vi "Next Pose.vi"(7 "Step":dbl=25.0, 8 "Start":T1 format="%.3f", 11 "Goal":T1 format="%.3f") -> (0 "Pose":T1 format="%.3f", 3 "At Goal":bool)   [LabVIEW 2013]
uses:
  <vilib>/Analysis/Matrix/Datatypes/RealMatrix.ctl
  <vilib>/Analysis/baseanly.llb/Real Dot Product.vi
  <vilib>/Analysis/Matrix/Numeric/Conversions/Array To Matrix - RA2.vi
  <vilib>/Analysis/NI_AALBase.lvlib
  <vilib>/Analysis/Matrix/NI_Matrix.lvlib
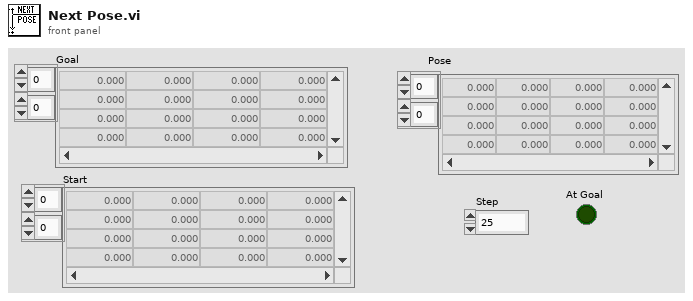
[diagram p1: front panel]
types:
  T1 = typedef "NI_Matrix.lvlib/RealMatrix.ctl" = dbl[][]
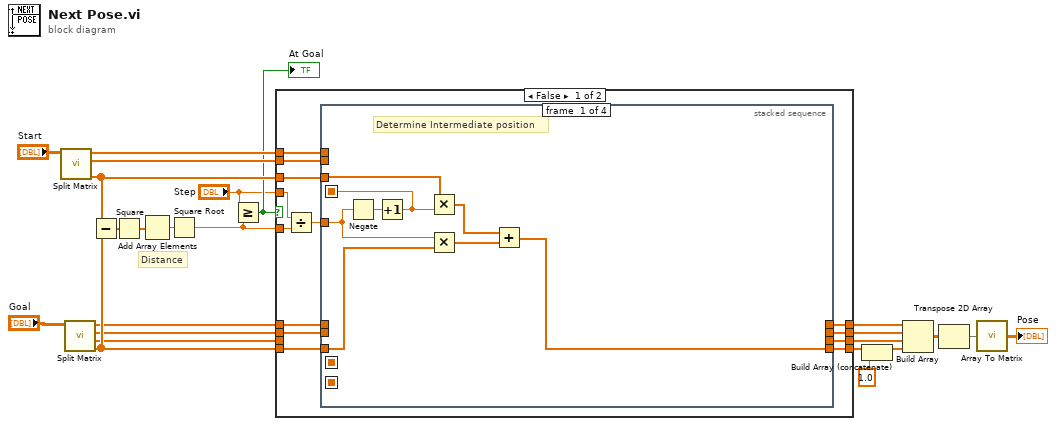
[diagram p0: block diagram]
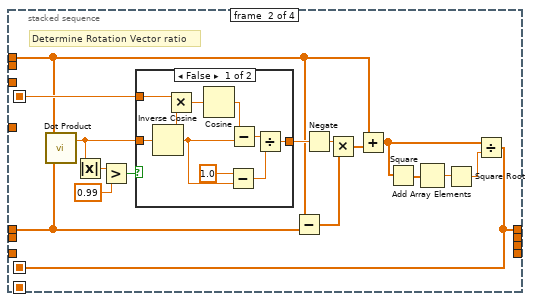
[diagram p2: hidden frame]
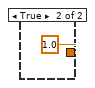
[diagram p3: hidden frame]
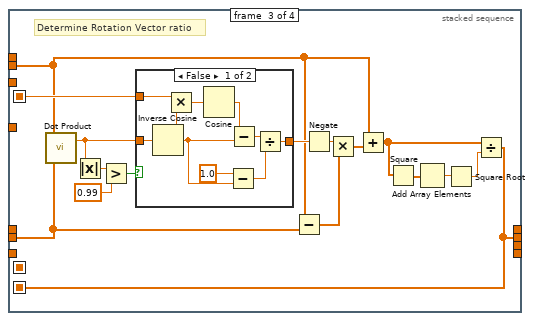
[diagram p4: hidden frame]
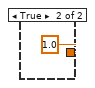
[diagram p5: hidden frame]
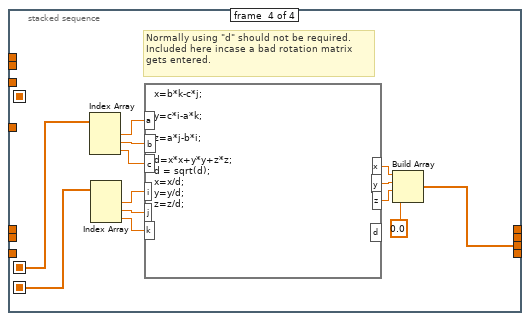
[diagram p6: hidden frame]
diagram:
  # "Distance"
  n1 = call "Split Matrix.vi"("Current"="Start") -> ("Position"=w21:dbl[], "Approach"=w17:dbl[], "Normal"=w18:dbl[])  [unwired: 7 in, 1 out]
  n2 = call "Split Matrix.vi"("Current"="Goal") -> ("Position"=w20:dbl[], "Tangent"=w14:dbl[], "Approach"=w15:dbl[], "Normal"=w16:dbl[])  [unwired: 7 in]
  n3 = Subtract ("Subtract.vi")(x=w21, y=w20) -> (x-y=w22:dbl[])
  n4 = Square(x=w22) -> (x^2=w23:dbl[])
  n5 = Add Array Elements(numeric array=w23) -> (sum=w24:dbl)
  n6 = Square Root(x=w24) -> (sqrt(x)=w4:dbl)
  n7 = Greater Or Equal?(x="Step", y=w4) -> (x >= y?=w6:bool)
  "At Goal" <- w6
  n8 = case shown="False" w6 {
    tunnel: w4 -> [w37 _]
    tunnel: "Step" -> [w35 _]
    tunnel: w20 -> [w34 w114]
    tunnel: w21 -> [w33 _]
    tunnel: [w32 w114] -> w2
    tunnel: w18 -> [w31 _]
    tunnel: w17 -> [w30 _]
    tunnel: w16 -> [w29 w113]
    tunnel: w15 -> [w28 w112]
    tunnel: [w27 w113] -> w11
    tunnel: [w26 w112] -> w12
    tunnel: w14 -> [_ w111]
    tunnel: [w25 w111] -> w13
    frame False {
      n9 = Divide(x=w35, y=w37) -> (x/y=w36:dbl)
      n10 = stacked-sequence {
        seq-local: [w39 _ _ _] -> [_ w61 w87 _]
        seq-local: [_ w46 _ _] -> [_ _ _ w98]
        seq-local: [_ _ w72 _] -> [_ _ _ w99]
        tunnel: w36 -> [w43 _ _ _]
        tunnel: w34 -> [w45 _ _ _]
        tunnel: w33 -> [w44 _ _ _]
        tunnel: [w38 _ _ _] -> w32
        tunnel: w31 -> [_ w51 _ _]
        tunnel: w30 -> [_ _ w73 _]
        tunnel: w29 -> [_ w56 _ _]
        tunnel: w28 -> [_ _ w74 _]
        tunnel: [_ w46 _ _] -> w27
        tunnel: [_ _ w72 _] -> w26
        tunnel: [_ _ _ w107] -> w25
        frame #0 {
          # "Determine Intermediate position"
          n11 = Negate(x=w43) -> (-x=w40:dbl)
          n12 = Increment(x=w40) -> (x+1=w39:dbl)
          n13 = Multiply ("Multiply.vi")(x=w44, y=w39) -> (x*y=w42:dbl[])
          n14 = Multiply ("Multiply.vi")(x=w43, y=w45) -> (x*y=w41:dbl[])
          n15 = Add ("Add.vi")(x=w42, y=w41) -> (x+y=w38:dbl[])
        }
        frame #1 {
          # "Determine Rotation Vector ratio"
          n16 = call-poly <vilib>:"Dot Product.vi"("Y Vector"=w56, "X Vector"=w51) -> ("X * Y"=w60:dbl)  [unwired: 1 out]
          n17 = Absolute Value(x=w60) -> (abs(x)=w59:dbl)
          n18 = Greater?(x=w59, y=0.99) -> (0:w57:bool)
          n19 = case shown="False" w57 {
            tunnel: w61 -> [w70 _]
            tunnel: w60 -> [w69 _]
            tunnel: [w62 1.0] -> w55
            frame False {
              n20 = Inverse Cosine(1:w69) -> (0:w66:dbl)
              n21 = Multiply(x=w70, y=w66) -> (x*y=w68:dbl)
              n22 = Cosine(x=w68) -> (cos(x)=w67:dbl)
              n23 = Subtract(x=1.0, y=w66) -> (x-y=w63:dbl)
              n24 = Subtract(x=w67, y=w66) -> (x-y=w64:dbl)
              n25 = Divide(x=w64, y=w63) -> (x/y=w62:dbl)
            }
            frame True {
            }
          }
          n26 = Subtract(x=w51, y=w56) -> (x-y=w54:dbl[])
          n27 = Negate(x=w55) -> (-x=w53:dbl)
          n28 = Multiply(x=w53, y=w54) -> (x*y=w52:dbl[])
          n29 = Add(x=w51, y=w52) -> (x+y=w47:dbl[])
          n30 = Square(x=w47) -> (x^2=w50:dbl[])
          n31 = Add Array Elements(numeric array=w50) -> (sum=w49:dbl)
          n32 = Square Root(x=w49) -> (sqrt(x)=w48:dbl)
          n33 = Divide(x=w47, y=w48) -> (x/y=w46:dbl[])
        }
        frame #2 {
          # "Determine Rotation Vector ratio"
          n34 = call-poly <vilib>:"Dot Product.vi"("Y Vector"=w74, "X Vector"=w73) -> ("X * Y"=w86:dbl)  [unwired: 1 out]
          n35 = Absolute Value(x=w86) -> (abs(x)=w85:dbl)
          n36 = Greater?(x=w85, y=0.99) -> (0:w83:bool)
          n37 = case shown="False" w83 {
            tunnel: w87 -> [w96 _]
            tunnel: w86 -> [w95 _]
            tunnel: [w88 1.0] -> w82
            frame False {
              n38 = Inverse Cosine(1:w95) -> (0:w92:dbl)
              n39 = Multiply(x=w96, y=w92) -> (x*y=w94:dbl)
              n40 = Cosine(x=w94) -> (cos(x)=w93:dbl)
              n41 = Subtract(x=1.0, y=w92) -> (x-y=w89:dbl)
              n42 = Subtract(x=w93, y=w92) -> (x-y=w90:dbl)
              n43 = Divide(x=w90, y=w89) -> (x/y=w88:dbl)
            }
            frame True {
            }
          }
          n44 = Subtract(x=w73, y=w74) -> (x-y=w81:dbl[])
          n45 = Negate(x=w82) -> (-x=w80:dbl)
          n46 = Multiply(x=w80, y=w81) -> (x*y=w79:dbl[])
          n47 = Add(x=w73, y=w79) -> (x+y=w75:dbl[])
          n48 = Square(x=w75) -> (x^2=w78:dbl[])
          n49 = Add Array Elements(numeric array=w78) -> (sum=w77:dbl)
          n50 = Square Root(x=w77) -> (sqrt(x)=w76:dbl)
          n51 = Divide(x=w75, y=w76) -> (x/y=w72:dbl[])
        }
        frame #3 {
          # "Normally using \"d\" should not be required.\nIncluded here incase a bad rotation matrix\ngets entered."
          n52 = Index Array(array=w98) -> (element #1=w106:dbl, element #2=w105:dbl, element #3=w104:dbl)  [unwired: 3 in]
          n53 = Index Array(array=w99) -> (element #1=w103:dbl, element #2=w102:dbl, element #3=w101:dbl)  [unwired: 3 in]
          n54 = formula code="x=b*k-c*j;\n\ny=c*i-a*k;\n\nz=a*j-b*i;\n\nd=x*x+y*y+z*z;\nd = sqrt(d);\nx=x/d;\ny=y/d;\nz=z/d;"("a"=w106, "b"=w105, "c"=w104, "i"=w103, "j"=w102, "k"=w101) -> ("x"=w109:dbl, "y"=w110:dbl, "z"=w108:dbl)  [unwired: 1 out]
          n55 = Build Array(w109, w110, w108, 0.0 ("element")) -> (w107:dbl[])
        }
      }
    }
    frame True {
    }
  }
  n56 = Build Array (concatenate)(w2, 1.0) -> (w1:dbl[])
  n57 = Build Array(w11, w12, w13, w1) -> (w10:dbl[][])
  n58 = Transpose 2D Array(2D array=w10) -> (transposed array=w9:dbl[][])
  n59 = call-poly <vilib>:"Array To Matrix.vi"("Real 2D Array"=w9) -> ("Real Matrix"=→"Pose":T1)
